vi "Einheit hinzufuegen.vi"(10 "Einheit":string, 11 "Eingang":string[](array[string])) -> (3 "Ausgang":string[](array[string]))   [LabVIEW 2020, in "EPA 1065.lvlib" / "ARN Test 1065-305.lvlib"]
uses:
  ARN Test 1065-305.lvlib
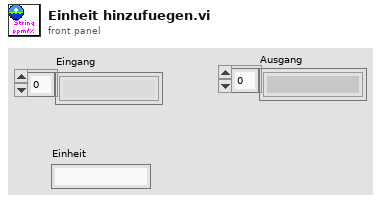
[diagram p1: front panel]
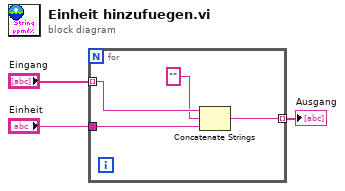
[diagram p0: block diagram]
diagram:
  n1 = for {
    tunnel: "Eingang" -> [w7] mode=indexing
    tunnel: "Einheit" -> [w5]
    tunnel: [w4] -> w1 mode=indexing
    n2 = Concatenate Strings(w7, "" ("String"), w5) -> (w4:string)
  }
  "Ausgang" <- w1
